vi "QuVI_3D Axis.vi"(6 "Character Size":sgl=0.5, 7 "Color":T1={"Red"=1.0, "Green"=0.0, "Blue"=0.0, "Alpha"=1.0}, 8 "error in (no error)":errorcluster, 9 "Radius":sgl=0.01, 10 "Length":sgl=2.0, 11 "Name":string="XYZ axis") -> (0 "error out":errorcluster, 3 "New Object Refnum":refnum<vi>)   [LabVIEW 2020]
uses:
  <vilib>/Utility/miscctls.llb/LVSceneTextAlignment.ctl
  <vilib>/picture/3D Picture Control/Object/Create Object (name).vi
  <vilib>/picture/3D Picture Control/Object/Create Object (drawable).vi
  <vilib>/picture/3D Picture Control/Object/Add Object (no reference).vi
  <vilib>/picture/3D Picture Control/NI_3D Picture Control.lvlib
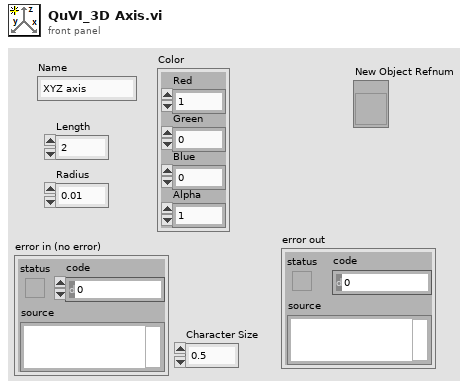
[diagram p1: front panel]
types:
  T1 = cluster{"Red":sgl, "Green":sgl, "Blue":sgl, "Alpha":sgl}
  T2 = typedef "LVSceneTextAlignment.ctl" = cluster{"Horizontal Alignment":enum8{"Left", "Right", "Center"}, "Vertical Alignment":enum8{"Top", "Bottom", "Center", "Base Line", "Bottom Base Line"}}
  T3 = cluster{"Alignment":T2, "Axis Alignment":enum8{"X-Y", "Y-Z", "X-Z", "Reversed X-Y", "Reversed Y-Z", "Reversed X-Z", "Screen"}, "Vertical?":bool, "Wrap Distance":sgl}
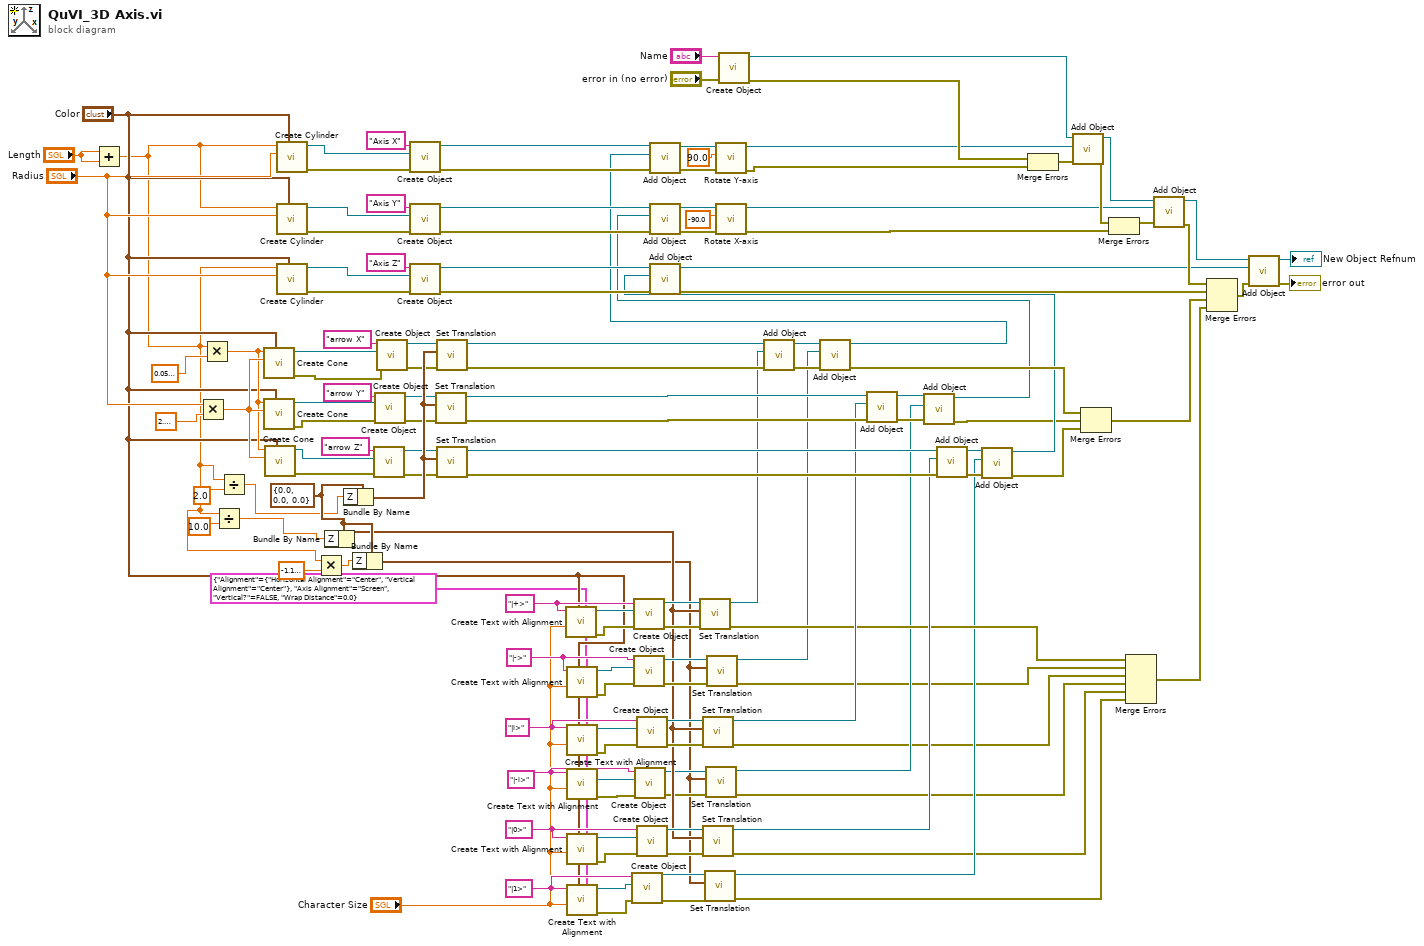
[diagram p0: block diagram]
diagram:
  w19 = "|1>" ("text")
  w25 = "|-i>" ("text")
  w48 = "|->" ("text")
  w64 = "|0>" ("text")
  w69 = "|i>" ("text")
  w5 = T3 {"Alignment"={"Horizontal Alignment"=enum."Center", "Vertical Alignment"=enum."Center"}, "Axis Alignment"=enum."Screen", "Vertical?"=FALSE, "Wrap Distance"=0.0} ("Font options")
  w58 = "|+>" ("text")
  w41 = cluster{"X":sgl, "Y":sgl, "Z":sgl} {"X"=0.0, "Y"=0.0, "Z"=0.0} ("Translation")
  n1 = Add(x="Length", y="Length") -> (x+y=w1:sgl)
  n2 = Multiply(x="Radius", y=sgl 2.2) -> (x*y=w131:sgl)
  n3 = Multiply(x=w1, y=sgl 0.05) -> (x*y=w130:sgl)
  n4 = Divide(x=w1, y=sgl 10.0 ("x")) -> (x/y=w2:sgl)
  n5 = Divide(x=w1, y=sgl 2.0 ("x")) -> (x/y=w3:sgl)
  n6 = call <vilib>:"Create Cone.vi"("Color"="Color", "Radius"=w131, "Height"=w130) -> ("error out"=w129:errorcluster, "New Cone Refnum"=w112:refnum<vi>)  [unwired: 7 in]
  n7 = call <vilib>:"Create Cone.vi"("Color"="Color", "Radius"=w131, "Height"=w130) -> ("error out"=w135:errorcluster, "New Cone Refnum"=w133:refnum<vi>)  [unwired: 7 in]
  n8 = call <vilib>:"Create Cone.vi"("Color"="Color", "Radius"=w131, "Height"=w130) -> ("error out"=w134:errorcluster, "New Cone Refnum"=w132:refnum<vi>)  [unwired: 7 in]
  n9 = call <vilib>:"Create Cylinder.vi"("Color"="Color", "Radius"="Radius", "Height"=w1) -> ("error out"=w89:errorcluster, "New Cylinder Refnum"=w83:refnum<vi>)  [unwired: 7 in]
  n10 = call <vilib>:"Create Cylinder.vi"("Color"="Color", "Radius"="Radius", "Height"=w1) -> ("error out"=w90:errorcluster, "New Cylinder Refnum"=w81:refnum<vi>)  [unwired: 7 in]
  n11 = call <vilib>:"Create Cylinder.vi"("Color"="Color", "Radius"="Radius", "Height"=w1) -> ("error out"=w91:errorcluster, "New Cylinder Refnum"=w82:refnum<vi>)  [unwired: 7 in]
  n12 = Multiply(x=w1, y=sgl -1.1) -> (x*y=w35:sgl)
  n13 = Bundle By Name(cluster=w41, "Z"=w2) -> (w40:cluster{"X":sgl, "Y":sgl, "Z":sgl})
  n14 = Bundle By Name(cluster=w41, "Z"=w3) -> (w114:cluster{"X":sgl, "Y":sgl, "Z":sgl})
  n15 = Bundle By Name(cluster=w41, "Z"=w35) -> (w14:cluster{"X":sgl, "Y":sgl, "Z":sgl})
  n16 = call-poly <vilib>:"Create Object.vi"("error in (no error)"=w134, "Geometry"=w132, "Name"="arrow Z") -> ("error out"=w111:errorcluster, "Scene:New Object"=w110:refnum<vi>)  [unwired: 7 in]
  n17 = call-poly <vilib>:"Create Object.vi"("error in (no error)"=w135, "Geometry"=w133, "Name"="arrow Y") -> ("error out"=w106:errorcluster, "Scene:New Object"=w107:refnum<vi>)  [unwired: 7 in]
  n18 = call-poly <vilib>:"Create Object.vi"("error in (no error)"=w129, "Geometry"=w112, "Name"="arrow X") -> ("error out"=w100:errorcluster, "Scene:New Object"=w99:refnum<vi>)  [unwired: 7 in]
  n19 = call-poly <vilib>:"Create Object.vi"("error in (no error)"=w89, "Geometry"=w83, "Name"="Axis X") -> ("error out"=w116:errorcluster, "Scene:New Object"=w103:refnum<vi>)  [unwired: 7 in]
  n20 = call-poly <vilib>:"Create Object.vi"("error in (no error)"=w90, "Geometry"=w81, "Name"="Axis Y") -> ("error out"=w127:errorcluster, "Scene:New Object"=w108:refnum<vi>)  [unwired: 7 in]
  n21 = call-poly <vilib>:"Create Object.vi"("error in (no error)"=w91, "Geometry"=w82, "Name"="Axis Z") -> ("error out"=w115:errorcluster, "Scene:New Object"=w113:refnum<vi>)  [unwired: 7 in]
  n22 = call <vilib>:"Set Translation.vi"("error in (no error)"=w106, "Translation"=w114, "Scene Object"=w107) -> ("error out"=w124:errorcluster, "Translated Object"=w118:refnum<vi>)  [unwired: 7 in]
  n23 = call <vilib>:"Set Translation.vi"("error in (no error)"=w100, "Translation"=w114, "Scene Object"=w99) -> ("error out"=w123:errorcluster, "Translated Object"=w39:refnum<vi>)  [unwired: 7 in]
  n24 = call <vilib>:"Set Translation.vi"("error in (no error)"=w111, "Translation"=w114, "Scene Object"=w110) -> ("error out"=w122:errorcluster, "Translated Object"=w119:refnum<vi>)  [unwired: 7 in]
  n25 = call <vilib>:"Create Text with Alignment.vi"("Font Options"=w5, "Color"="Color", "Character Size"="Character Size", "Text"=w58) -> ("error out"=w57:errorcluster, "New Text Refnum"=w71:refnum<vi>)  [unwired: 6 in]
  n26 = call <vilib>:"Create Text with Alignment.vi"("Font Options"=w5, "Color"="Color", "Character Size"="Character Size", "Text"=w48) -> ("error out"=w46:errorcluster, "New Text Refnum"=w47:refnum<vi>)  [unwired: 6 in]
  n27 = call <vilib>:"Create Text with Alignment.vi"("Font Options"=w5, "Color"="Color", "Character Size"="Character Size", "Text"=w69) -> ("error out"=w61:errorcluster, "New Text Refnum"=w68:refnum<vi>)  [unwired: 6 in]
  n28 = call <vilib>:"Create Text with Alignment.vi"("Font Options"=w5, "Color"="Color", "Character Size"="Character Size", "Text"=w25) -> ("error out"=w23:errorcluster, "New Text Refnum"=w24:refnum<vi>)  [unwired: 6 in]
  n29 = call <vilib>:"Create Text with Alignment.vi"("Font Options"=w5, "Color"="Color", "Character Size"="Character Size", "Text"=w64) -> ("error out"=w63:errorcluster, "New Text Refnum"=w65:refnum<vi>)  [unwired: 6 in]
  n30 = call <vilib>:"Create Text with Alignment.vi"("Font Options"=w5, "Color"="Color", "Character Size"="Character Size", "Text"=w19) -> ("error out"=w17:errorcluster, "New Text Refnum"=w18:refnum<vi>)  [unwired: 6 in]
  n31 = call-poly <vilib>:"Create Object.vi"("error in (no error)"=w17, "Geometry"=w18, "Name"=w19) -> ("error out"=w16:errorcluster, "Scene:New Object"=w15:refnum<vi>)  [unwired: 7 in]
  n32 = call-poly <vilib>:"Create Object.vi"("error in (no error)"=w57, "Geometry"=w71, "Name"=w58) -> ("error out"=w59:errorcluster, "Scene:New Object"=w70:refnum<vi>)  [unwired: 7 in]
  n33 = call-poly <vilib>:"Create Object.vi"("error in (no error)"=w46, "Geometry"=w47, "Name"=w48) -> ("error out"=w45:errorcluster, "Scene:New Object"=w49:refnum<vi>)  [unwired: 7 in]
  n34 = call-poly <vilib>:"Create Object.vi"("error in (no error)"=w23, "Geometry"=w24, "Name"=w25) -> ("error out"=w21:errorcluster, "Scene:New Object"=w22:refnum<vi>)  [unwired: 7 in]
  n35 = call-poly <vilib>:"Create Object.vi"("error in (no error)"=w61, "Geometry"=w68, "Name"=w69) -> ("error out"=w60:errorcluster, "Scene:New Object"=w67:refnum<vi>)  [unwired: 7 in]
  n36 = call-poly <vilib>:"Create Object.vi"("error in (no error)"=w63, "Geometry"=w65, "Name"=w64) -> ("error out"=w62:errorcluster, "Scene:New Object"=w66:refnum<vi>)  [unwired: 7 in]
  n37 = call <vilib>:"Set Translation.vi"("error in (no error)"=w59, "Translation"=w40, "Scene Object"=w70) -> ("error out"=w56:errorcluster, "Translated Object"=w37:refnum<vi>)  [unwired: 7 in]
  n38 = call <vilib>:"Set Translation.vi"("error in (no error)"=w60, "Translation"=w40, "Scene Object"=w67) -> ("error out"=w10:errorcluster, "Translated Object"=w73:refnum<vi>)  [unwired: 7 in]
  n39 = call <vilib>:"Set Translation.vi"("error in (no error)"=w62, "Translation"=w40, "Scene Object"=w66) -> ("error out"=w8:errorcluster, "Translated Object"=w72:refnum<vi>)  [unwired: 7 in]
  n40 = call <vilib>:"Set Translation.vi"("error in (no error)"=w16, "Translation"=w14, "Scene Object"=w15) -> ("error out"=w12:errorcluster, "Translated Object"=w13:refnum<vi>)  [unwired: 7 in]
  n41 = call <vilib>:"Set Translation.vi"("error in (no error)"=w21, "Translation"=w14, "Scene Object"=w22) -> ("error out"=w9:errorcluster, "Translated Object"=w20:refnum<vi>)  [unwired: 7 in]
  n42 = call <vilib>:"Set Translation.vi"("error in (no error)"=w45, "Translation"=w14, "Scene Object"=w49) -> ("error out"=w11:errorcluster, "Translated Object"=w36:refnum<vi>)  [unwired: 7 in]
  n43 = call-poly <vilib>:"Create Object.vi"("error in (no error)"="error in (no error)", "Name"="Name") -> ("error out"=w92:errorcluster, "Scene:New Object"=w75:refnum<vi>)  [unwired: 8 in]
  n44 = call-poly <vilib>:"Add Object.vi"("error in (no error)"=w123, "New Object In"=w37, "Scene Object In"=w39) -> ("error out"=w44:errorcluster, "Scene Object Out"=w38:refnum<vi>)  [unwired: 7 in]
  n45 = call-poly <vilib>:"Add Object.vi"("error in (no error)"=w44, "New Object In"=w36, "Scene Object In"=w38) -> ("error out"=w43:errorcluster, "Scene Object Out"=w42:refnum<vi>)  [unwired: 7 in]
  n46 = call-poly <vilib>:"Add Object.vi"("error in (no error)"=w116, "New Object In"=w42, "Scene Object In"=w103) -> ("error out"=w117:errorcluster, "Scene Object Out"=w104:refnum<vi>)  [unwired: 7 in]
  n47 = call <vilib>:"Rotate Y-axis.vi"("error in (no error)"=w117, "angle"=90.0, "Scene Object In"=w104) -> ("error out"=w50:errorcluster, "Scene Object Out"=w51:refnum<vi>)  [unwired: 7 in]
  n48 = call-poly <vilib>:"Add Object.vi"("error in (no error)"=w124, "New Object In"=w73, "Scene Object In"=w118) -> ("error out"=w29:errorcluster, "Scene Object Out"=w28:refnum<vi>)  [unwired: 7 in]
  n49 = call-poly <vilib>:"Add Object.vi"("error in (no error)"=w29, "New Object In"=w20, "Scene Object In"=w28) -> ("error out"=w27:errorcluster, "Scene Object Out"=w26:refnum<vi>)  [unwired: 7 in]
  n50 = call-poly <vilib>:"Add Object.vi"("error in (no error)"=w127, "New Object In"=w26, "Scene Object In"=w108) -> ("error out"=w128:errorcluster, "Scene Object Out"=w109:refnum<vi>)  [unwired: 7 in]
  n51 = call <vilib>:"Rotate X-axis.vi"("error in (no error)"=w128, "angle"=-90.0, "Scene Object In"=w109) -> ("error out"=w53:errorcluster, "Scene Object Out"=w52:refnum<vi>)  [unwired: 7 in]
  n52 = call-poly <vilib>:"Add Object.vi"("error in (no error)"=w122, "New Object In"=w72, "Scene Object In"=w119) -> ("error out"=w32:errorcluster, "Scene Object Out"=w33:refnum<vi>)  [unwired: 7 in]
  n53 = call-poly <vilib>:"Add Object.vi"("error in (no error)"=w32, "New Object In"=w13, "Scene Object In"=w33) -> ("error out"=w30:errorcluster, "Scene Object Out"=w31:refnum<vi>)  [unwired: 7 in]
  n54 = call-poly <vilib>:"Add Object.vi"("error in (no error)"=w115, "New Object In"=w31, "Scene Object In"=w113) -> ("error out"=w54:errorcluster, "Scene Object Out"=w55:refnum<vi>)  [unwired: 7 in]
  n55 = Merge Errors(w92, w50) -> (w93:errorcluster)
  n56 = call-poly <vilib>:"Add Object.vi"("error in (no error)"=w93, "New Object In"=w51, "Scene Object In"=w75) -> ("error out"=w94:errorcluster, "Scene Object Out"=w76:refnum<vi>)  [unwired: 7 in]
  n57 = Merge Errors(w43, w27, w30) -> (w125:errorcluster)
  n58 = Merge Errors(w94, w53) -> (w95:errorcluster)
  n59 = Merge Errors(w56, w11, w10, w9, w8, w12) -> (w126:errorcluster)
  n60 = call-poly <vilib>:"Add Object.vi"("error in (no error)"=w95, "New Object In"=w52, "Scene Object In"=w76) -> ("error out"=w96:errorcluster, "Scene Object Out"=w77:refnum<vi>)  [unwired: 7 in]
  n61 = Merge Errors(w96, w54, w125, w126) -> (w97:errorcluster)
  n62 = call-poly <vilib>:"Add Object.vi"("error in (no error)"=w97, "New Object In"=w55, "Scene Object In"=w77) -> ("error out"=→"error out":errorcluster, "Scene Object Out"=→"New Object Refnum":refnum<vi>)  [unwired: 7 in]
